vi "To Start and Stop (frequency).vi"(4 "span":dbl[unit], 6 "center":dbl[unit]) -> (0 "stop":dbl[unit], 2 "start":dbl[unit])   [LabVIEW 2012]
doc: "Takes two frequencies that indicate the average (\"center\") and difference (\"span\") of a frequency range and returns the beginning and end of the range."
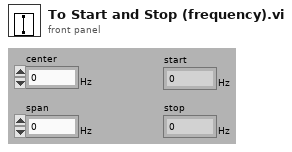
[diagram p1: front panel]
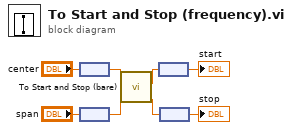
[diagram p0: block diagram]
diagram:
  n1 = node("center") -> (w6:dbl)
  n2 = node("span") -> (w5:dbl)
  n3 = call "To Start and Stop (bare).vi"("span"=w5, "center"=w6) -> ("stop"=w4:dbl, "start"=w3:dbl)  [unwired: 4 out]
  n4 = node(w3) -> (→"start":dbl[unit])
  n5 = node(w4) -> (→"stop":dbl[unit])
